vi "get and check exp config.vi"(0 "Working Directory In":path, 1 "App Name":string) -> (4 "Write To File":bool, 6 "Data File Prefix":string="data", 7 "Interval (ms)":u32=500, 9 "Resolution":u8, 10 "Graph History":i32=1000 min=0, 11 "SettlingFactor":u8, 13 "Device Config File Name":string, 14 "# Channels":i32=4, 16 "Disable Scaling":bool, 17 "Max File Size (Bytes)":i32=1048576, 18 "Channel Setup":T1={"+Ch"=["0", "1", "2", "3", "4", "5", "6", "7"], "-Ch"=["199", "199", "199", "199", "199", "199", "199", "199"], "Ranges"=[0, 0, 0, 0, 0, 0, 0, 0], "Scaling Equation"=["y=v0", "y=v1", "y=v2", "y=v3", "y=v4", "y=v5", "y=v6", "y=v7"], "Graph?"=[]} {"Ranges" items=["LJ_rgBIP10V", "LJ_rgBIP5V", "LJ_rgUNI5V", "LJ_rgUNI2P5V", "LJ_rgUNI1P25V", "LJ_rgBIP1V", "LJ_rgUNIP625V", "LJ_rgBIPP1V", "LJ_rgBIPP01V"]}, 19 "error out":errorcluster)   [LabVIEW 2020]
panel:
  out "Scan Rate (Hz)":dbl=500.0 format="%.3f"
  out "Device Config Path":path
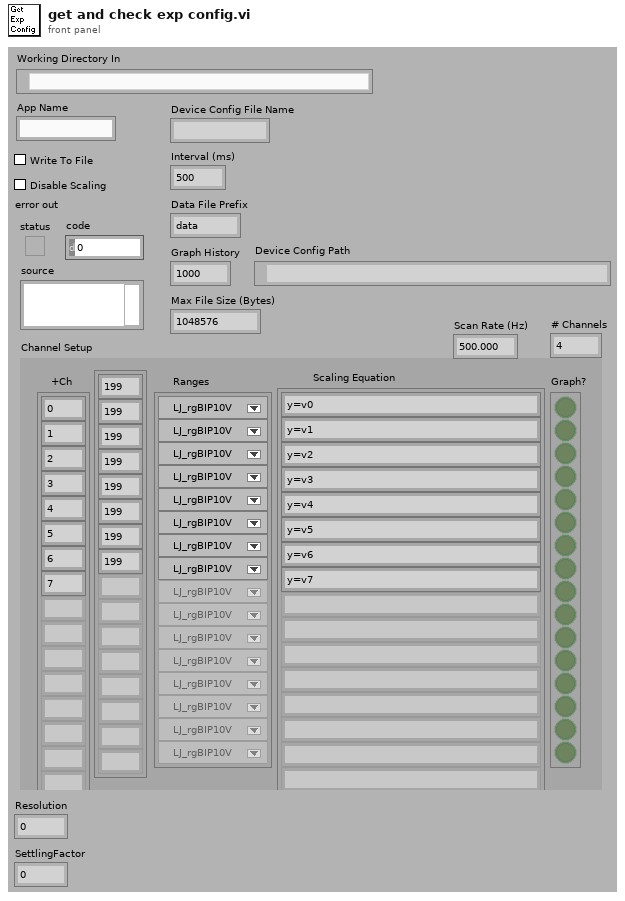
[diagram p1: front panel]
types:
  T1 = cluster{"+Ch":string[], "-Ch":string[], "Ranges":u16[], "Scaling Equation":string[], "Graph?":bool[]}
  T2 = enum16{"Left Button", "Center Button", "Right Button", "Window Close"}
  T3 = enum32{"existing file", "new file", "new or existing file", "existing dir", "new dir", "new or existing dir", "existing file (use LLBs)", "new file (use LLBs)", "new or existing file (use LLBs)", "new or existing file or directory (use LLBs)"}
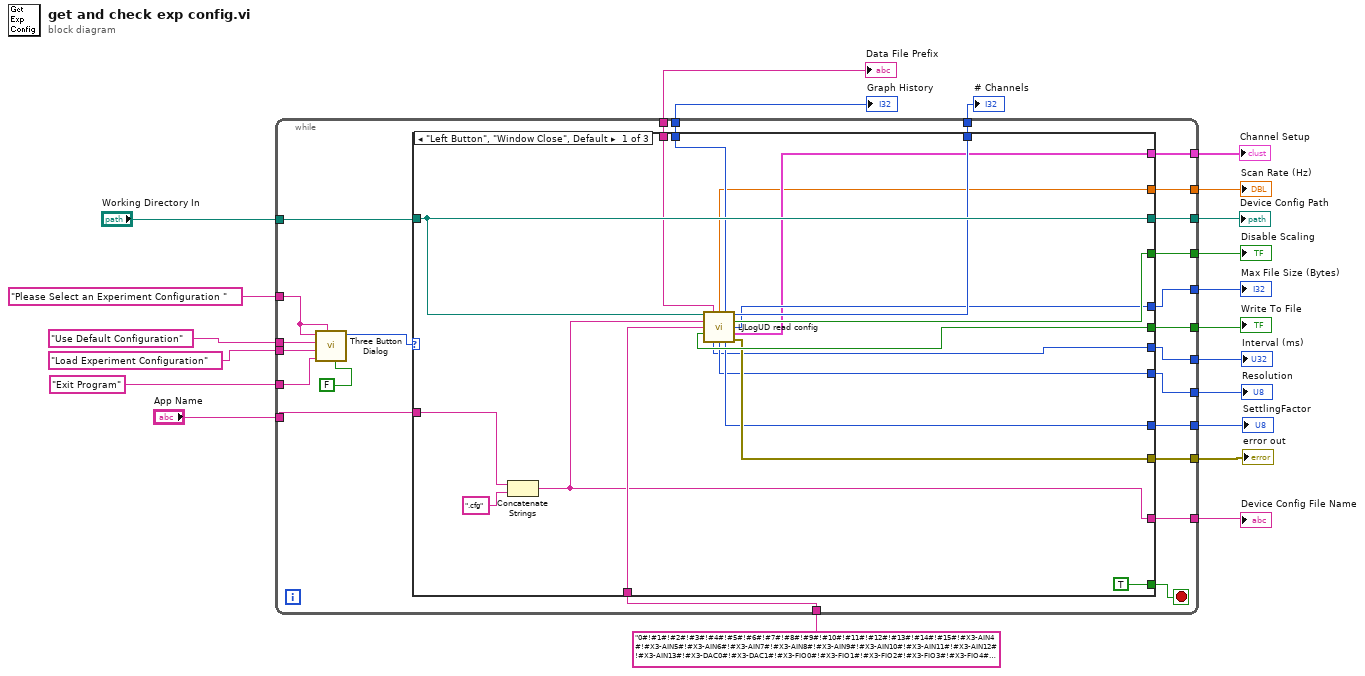
[diagram p0: block diagram]
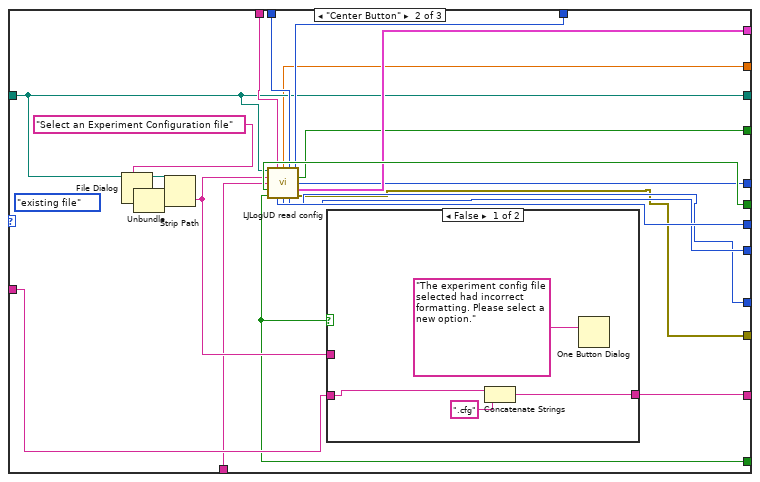
[diagram p2: hidden frame]
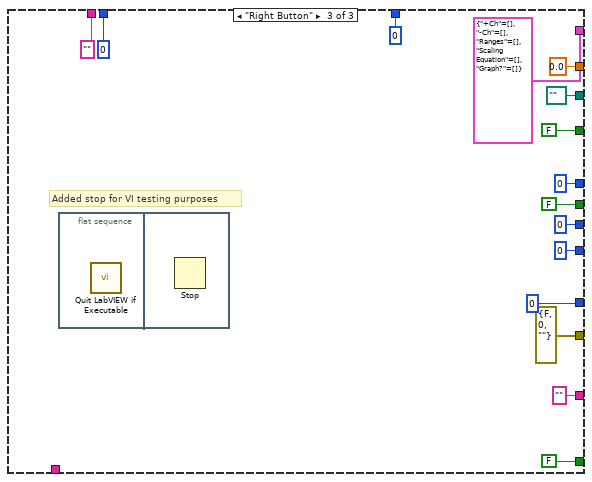
[diagram p4: hidden frame]
diagram:
  n1 = while {
    tunnel: "Working Directory In" -> [w45]
    tunnel: "App Name" -> [w44]
    tunnel: [w43] -> w19
    tunnel: [w42] -> w18
    tunnel: [w41] -> w17
    tunnel: [w40] -> w16
    tunnel: [w39] -> w15
    tunnel: [w38] -> w14
    tunnel: [w37] -> w13
    tunnel: [w36] -> w12
    tunnel: [w35] -> w11
    tunnel: [w34] -> w10
    tunnel: [w33] -> w9
    tunnel: "0#!#1#!#2#!#3#!#4#!#5#!#6#!#7#!#8#!#9#!#10#!#11#!#12#!#13#!#14#!#15#!#X3-AIN4#!#X3-AIN5#!#X3-AIN6#!#X3-AIN7#!#X3-AIN8#!#X3-AIN9#!#X3-AIN10#!#X3-AIN11#!#X3-AIN12#!#X3-AIN13#!#X3-DAC0#!#X3-DAC1#!#X3-FIO0#!#X3-FIO1#!#X3-FIO2#!#X3-FIO3#!#X3-FIO4#!#X3-FIO5#!#X3-FIO6#!#X3-FIO7#!#X4-AIN0#!#X4-AIN1#!#X4-AIN2#!#X4-AIN3#!#X4-AIN4#!#X4-AIN5#!#X4-AIN6#!#X4-AIN7#!#X4-AIN8#!#X4-AIN9#!#X4-AIN10#!#X4-AIN11#!#X4-AIN12#!#X4-AIN13#!#X4-DAC0#!#X4-DAC1#!#X4-FIO0#!#X4-FIO1#!#X4-FIO2#!#X4-FIO3#!#X4-FIO4#!#X4-FIO5#!#X4-FIO6#!#X4-FIO7#!#X5-AIN0#!#X5-AIN1#!#X5-AIN2#!#X5-AIN3#!#X5-AIN4#!#X5-AIN5#!#X5-AIN6#!#X5-AIN7#!#X5-AIN8#!#X5-AIN9#!#X5-AIN10#!#X5-AIN11#!#X5-AIN12#!#X5-AIN13#!#X5-DAC0#!#X5-DAC1#!#X5-FIO0#!#X5-FIO1#!#X5-FIO2#!#X5-FIO3#!#X5-FIO4#!#X5-FIO5#!#X5-FIO6#!#X5-FIO7#!#" -> [w32]
    tunnel: [w31] -> w7
    tunnel: [w30] -> w6
    tunnel: [w29] -> w5
    tunnel: "Use Default Configuration" ("F button name (\"Cancel\")") -> [w28]
    tunnel: "Load Experiment Configuration" ("T button name (\"OK\")") -> [w27]
    tunnel: "Exit Program" ("Right Button Text (\"Cancel\")") -> [w26]
    tunnel: "Please Select an Experiment Configuration " ("message") -> [w25]
    stop <- w23 stop-if-true
    n2 = call <vilib>:"Three Button Dialog.vi"("Allow user to close window? (TRUE)"=FALSE, "Window Title (\"\")"=w25, "Right Button Text (\"Cancel\")"=w26, "Center Button Text (\"No\")"=w27, "Left Button Text (\"Yes\")"=w28, "message"=w25) -> ("Which Button?"=w24:T2)  [unwired: 5 in]
    n3 = case shown="\"Left Button\", \"Window Close\", Default" w24 {
      tunnel: w45 -> [w58 w70 _]
      tunnel: w44 -> [w62 w82 _]
      tunnel: [w58 w70 path "" ("Working Directory In")] -> w43
      tunnel: [w61 w80 FALSE ("Write To File")] -> w42
      tunnel: [w48 w79 u32 0 ("Interval (ms)")] -> w41
      tunnel: [w57 w71 "" ("Data File Prefix")] -> w40
      tunnel: [w56 w72 0 ("Graph History")] -> w39
      tunnel: [w55 w73 0 ("# Channels")] -> w38
      tunnel: [w54 w74 FALSE ("Disable Scaling")] -> w37
      tunnel: [w53 w75 0 ("Max File Size (Bytes)")] -> w36
      tunnel: [w52 w76 T1 {"+Ch"=[], "-Ch"=[], "Ranges"=[], "Scaling Equation"=[], "Graph?"=[]} ("Channel Setup")] -> w35
      tunnel: w32 -> [w60 w68 _]
      tunnel: [w59 w81 "" ("name")] -> w34
      tunnel: [w51 w67 errorcluster {"status"=FALSE, "code"=0, "source"=""} ("error out")] -> w33
      tunnel: [w49 w78 u8 0 ("Resolution")] -> w31
      tunnel: [w50 w77 u8 0 ("SettlingFactor")] -> w30
      tunnel: [w47 w66 0.0 ("Scan Rate (Hz)")] -> w29
      tunnel: [TRUE ("Good Config File") w65 FALSE ("Good Config File")] -> w23
      frame "Left Button", "Window Close", Default {
        n4 = Concatenate Strings(w62, ".cfg" ("filename")) -> (w59:string)
        n5 = call "LJLogUD read config.vi"("Working Directory"=w58, "filename"=w59, "ChP Default"=w60) -> ("Data File Prefix"=w57:string, "Scan Rate (Hz)"=w47:dbl, "Graph History"=w56:i32, "# Channels"=w55:i32, "Disable Scaling"=w54:bool, "Max File Size (Bytes)"=w53:i32, "Write To File"=w61:bool, "Channel Setup"=w52:T1, "Interval (ms)"=w48:u32, "Resolution"=w49:u8, "SettlingFactor"=w50:u8, "error out"=w51:errorcluster)  [unwired: 1 out]
      }
      frame "Center Button" {
        (unwired) T3."existing file" ("select mode (2)")
        n6 = File Dialog(7:"Select an Experiment Configuration file" ("Substring"), 11:w70) -> (0:w64:errorcluster, 3:w83:path)  [unwired: 5 in, 2 out]
        n7 = Unbundle(w64) -> ()  [unwired: 3 out]
        n8 = Strip Path(path=w83) -> (name=w69:string)  [unwired: 1 out]
        n9 = call "LJLogUD read config.vi"("Working Directory"=w70, "filename"=w69, "ChP Default"=w68) -> ("Data File Prefix"=w71:string, "Scan Rate (Hz)"=w66:dbl, "Graph History"=w72:i32, "# Channels"=w73:i32, "Disable Scaling"=w74:bool, "Max File Size (Bytes)"=w75:i32, "Write To File"=w80:bool, "Channel Setup"=w76:T1, "Good Config File"=w65:bool, "Interval (ms)"=w79:u32, "Resolution"=w78:u8, "SettlingFactor"=w77:u8, "error out"=w67:errorcluster)
        n10 = case shown="False" w65 {
          tunnel: w82 -> [w86 _]
          tunnel: [w85 w89] -> w81
          tunnel: w69 -> [_ w89]
          frame False {
            n11 = Concatenate Strings(w86, ".cfg" ("string")) -> (w85:string)
            n12 = One Button Dialog(message="The experiment config file selected had incorrect formatting. Please select a new option.") -> ()  [unwired: 1 in, 1 out]
          }
          frame True {
          }
        }
      }
      frame "Right Button" {
        # "Added stop for VI testing purposes"
        n13 = flat-sequence {
          frame #0 {
            n14 = call "Quit LabVIEW if Executable.vi"() -> ()  [unwired: 1 in]
          }
          frame #1 {
            n15 = Stop() -> ()  [unwired: 1 in]
          }
        }
      }
    }
  }
  "Device Config Path" <- w19
  "Device Config File Name" <- w10
  "error out" <- w9
  "Interval (ms)" <- w17
  "Write To File" <- w18
  "Data File Prefix" <- w16
  "Graph History" <- w15
  "# Channels" <- w14
  "Disable Scaling" <- w13
  "Max File Size (Bytes)" <- w12
  "Channel Setup" <- w11
  "Scan Rate (Hz)" <- w5
  "Resolution" <- w7
  "SettlingFactor" <- w6
